vi "Unit Test - copy and Replace State.vi"() -> (3 "Array":T1(array[cluster])=[{"state"="Idle", "error out"={"status"=FALSE, "code"=0, "source"=""}, "Execution:State"=enum."Idle"}, {"state"="CSM Documentation", "error out"={"status"=FALSE, "code"=0, "source"=""}, "Execution:State"=enum."Idle"}, {"state"="VI Reference", "error out"={"status"=FALSE, "code"=0, "source"=""}, "Execution:State"=enum."Idle"}, {"state"="Error Handler", "error out"={"status"=FALSE, "code"=0, "source"=""}, "Execution:State"=enum."Bad"}, {"state"="Critical Error", "error out"={"status"=FALSE, "code"=0, "source"=""}, "Execution:State"=enum."Idle"}, {"state"="Target Timeout Error", "error out"={"status"=FALSE, "code"=0, "source"=""}, "Execution:State"=enum."Idle"}, {"state"="Target Error", "error out"={"status"=FALSE, "code"=0, "source"=""}, "Execution:State"=enum."Idle"}, {"state"="Async Response", "error out"={"status"=FALSE, "code"=0, "source"=""}, "Execution:State"=enum."Idle"}, {"state"="Response", "error out"={"status"=FALSE, "code"=0, "source"=""}, "Execution:State"=enum."Idle"}, {"state"="Async Message Posted", "error out"={"status"=FALSE, "code"=0, "source"=""}, "Execution:State"=enum."Idle"}, {"state"="Initialize Core Data", "error out"={"status"=FALSE, "code"=0, "source"=""}, "Execution:State"=enum."Idle"}, {"state"="Exit", "error out"={"status"=FALSE, "code"=0, "source"=""}, "Execution:State"=enum."Idle"}, {"state"="Data: Initialize", "error out"={"status"=FALSE, "code"=0, "source"=""}, "Execution:State"=enum."Idle"}, {"state"="Data: Update Indicators", "error out"={"status"=FALSE, "code"=0, "source"=""}, "Execution:State"=enum."Idle"}, {"state"="Data: Cleanup", "error out"={"status"=FALSE, "code"=0, "source"=""}, "Execution:State"=enum."Idle"}, {"state"="Macro: Initialize", "error out"={"status"=FALSE, "code"=0, "source"=""}, "Execution:State"=enum."Idle"}, {"state"="Macro: Exit", "error out"={"status"=FALSE, "code"=0, "source"=""}, "Execution:State"=enum."Idle"}, {"state"="API: API1", "error out"={"status"=FALSE, "code"=0, "source"=""}, "Execution:State"=enum."Idle"}, {"state"="API: API2", "error out"={"status"=FALSE, "code"=0, "source"=""}, "Execution:State"=enum."Idle"}, {"state"="Action: action1", "error out"={"status"=FALSE, "code"=0, "source"=""}, "Execution:State"=enum."Idle"}, {"state"="Action: action2", "error out"={"status"=FALSE, "code"=0, "source"=""}, "Execution:State"=enum."Idle"}])   [LabVIEW 2017, in "testcase-csmhelper.lvclass"]
uses:
  testcase-csmhelper.lvclass
  src/user.lib/_NEVSTOP/Communicable State Machine(CSM)/_csmHelper/CSM-Helper.lvclass/CSM-Helper.ctl
  src/user.lib/_NEVSTOP/Communicable State Machine(CSM)/_csmHelper/Properties/Read VI Ref.vi
  src/user.lib/_NEVSTOP/Communicable State Machine(CSM)/_csmHelper/API/Create From VI Reference.vi
  src/user.lib/_NEVSTOP/Communicable State Machine(CSM)/_csmHelper/API/Open Block Diagram.vi
  src/user.lib/_NEVSTOP/Communicable State Machine(CSM)/_csmHelper/Properties/Read User-Defined States.vi
  src/user.lib/_NEVSTOP/Communicable State Machine(CSM)/_csmHelper/API/Start Undo.vi
  src/user.lib/_NEVSTOP/Communicable State Machine(CSM)/_csmHelper/API/Copy State.vi
  src/user.lib/_NEVSTOP/Communicable State Machine(CSM)/_csmHelper/API/Stop Undo.vi
  src/user.lib/_NEVSTOP/Communicable State Machine(CSM)/_csmHelper/API/Undo.vi
  src/user.lib/_NEVSTOP/Communicable State Machine(CSM)/_csmHelper/API/Destroy.vi
  src/user.lib/_NEVSTOP/Communicable State Machine(CSM)/_csmHelper/CSM-Helper.lvclass
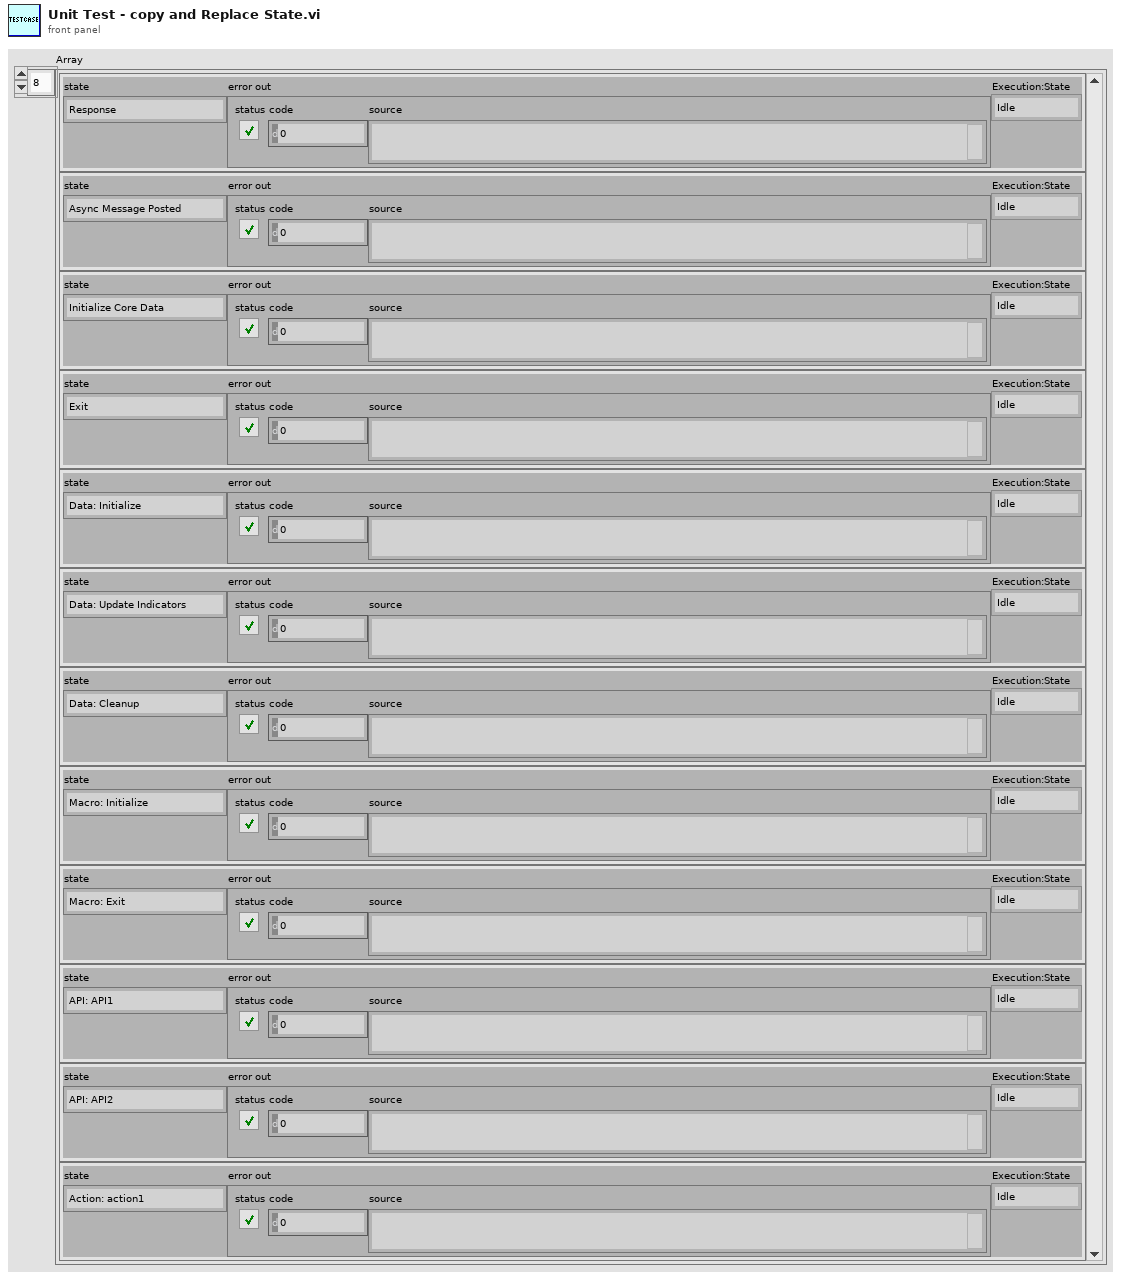
[diagram p1: front panel]
types:
  T1 = cluster{"state":string, "error out":errorcluster, "Execution:State":enum32{"Bad", "Idle", "Run top level", "Running"}}[]
  T2 = enum32{"Bad", "Idle", "Run top level", "Running"}
  T3 = cluster{string, "error out":errorcluster, "Exec.State":enum32{"Bad", "Idle", "Run top level", "Running"}}
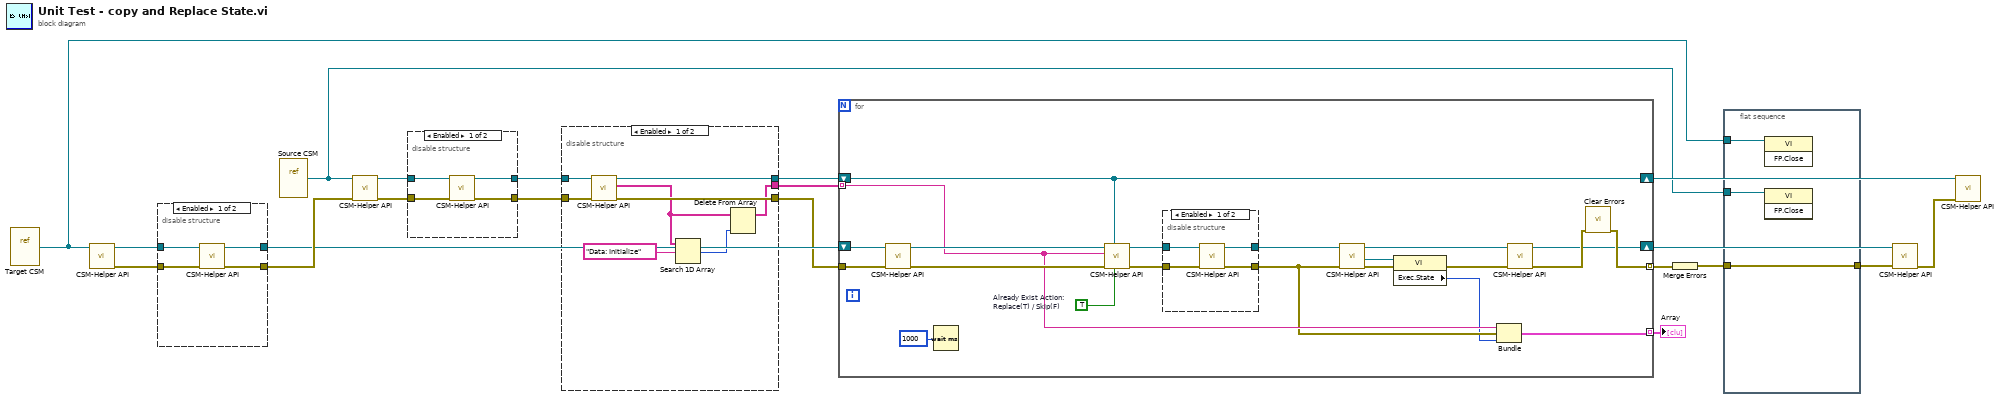
[diagram p0: block diagram]
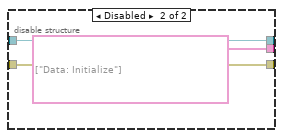
[diagram p2: hidden frame]
diagram:
  n1 = vi-ref "Target CSM.vi"() -> (w2:refnum<vi>)
  n2 = call-poly "CSM-Helper API.vi"("VI"=w2) -> ("error out"=w18:errorcluster, "CSM-Helper.lvclass"=w17:refnum<class "CSM-Helper.lvclass">)  [unwired: 9 in]
  n3 = disable-structure shown="Enabled" {
    disable-tunnel: w18 -> [w24 w26]
    disable-tunnel: w17 -> [w23 w25]
    disable-tunnel: [w22 w26] -> w12
    disable-tunnel: [w21 w25] -> w11
    frame Enabled {
      n4 = call-poly "CSM-Helper API.vi"("error in (no error)"=w24, "CSM-Helper in"=w23) -> ("error out"=w22:errorcluster, "CSM-Helper out"=w21:refnum<class "CSM-Helper.lvclass">)  [unwired: 8 in]
    }
    frame Disabled {
    }
  }
  n5 = vi-ref "Source CSM.vi"() -> (w1:refnum<vi>)
  n6 = call-poly "CSM-Helper API.vi"("error in (no error)"=w12, "VI"=w1) -> ("error out"=w15:errorcluster, "CSM-Helper.lvclass"=w16:refnum<class "CSM-Helper.lvclass">)  [unwired: 8 in]
  n7 = disable-structure shown="Enabled" {
    disable-tunnel: w16 -> [w30 w31]
    disable-tunnel: w15 -> [w29 w32]
    disable-tunnel: [w28 w32] -> w14
    disable-tunnel: [w27 w31] -> w13
    frame Enabled {
      n8 = call-poly "CSM-Helper API.vi"("error in (no error)"=w29, "CSM-Helper in"=w30) -> ("error out"=w28:errorcluster, "CSM-Helper out"=w27:refnum<class "CSM-Helper.lvclass">)  [unwired: 8 in]
    }
    frame Disabled {
    }
  }
  n9 = disable-structure shown="Enabled" {
    disable-tunnel: w14 -> [w40 w42]
    disable-tunnel: w13 -> [w39 w43]
    disable-tunnel: [w38 w42] -> w10
    disable-tunnel: [w37 w43] -> w9
    disable-tunnel: [w34 string[] ["Data: Initialize"] ("Value")] -> w6
    frame Enabled {
      n10 = call-poly "CSM-Helper API.vi"("error in (no error)"=w40, "CSM-Helper in"=w39) -> ("error out"=w38:errorcluster, "Array"=w35:string[], "CSM-Helper out"=w37:refnum<class "CSM-Helper.lvclass">)  [unwired: 7 in]
      n11 = Search 1D Array(1D array=w35, element="Data: Initialize") -> (index of element=w33:i32)  [unwired: 1 in]
      n12 = Delete From Array(array=w35, index=w33) -> (array with subset deleted=w34:string[])  [unwired: 1 in, 1 out]
    }
    frame Disabled {
    }
  }
  n13 = for {
    shift-right: [w52] -> w20
    shift-left: w11 -> [w63]
    shift-right: [w58] -> w7
    shift-left: w9 -> [w58]
    tunnel: w6 -> [w56] mode=indexing
    tunnel: w10 -> [w62]
    tunnel: [w57] -> w19 mode=indexing
    tunnel: [w55] -> w5 mode=indexing
    w44 = TRUE  # Already Exist Action: Replace(T) / Skip(F)
    n14 = call-poly "CSM-Helper API.vi"("error in (no error)"=w62, "CSM-Helper in"=w63) -> ("error out"=w61:errorcluster, "CSM-Helper out"=w60:refnum<class "CSM-Helper.lvclass">)  [unwired: 8 in]
    n15 = Wait (ms)(milliseconds to wait=u32 1000) -> ()  [unwired: 1 out]
    n16 = call-poly "CSM-Helper API.vi"("Already Exist Action:\nReplace(T) / Skip(F)"=w44, "SourceCSM"=w58, "error in (no error)"=w61, "Case"=w56, "CSM-Helper.lvclass"=w60) -> ("error out"=w59:errorcluster, "CSM-Helper out 2"=w64:refnum<class "CSM-Helper.lvclass">)  [unwired: 5 in]
    n17 = disable-structure shown="Enabled" {
      disable-tunnel: [w68 w70] -> w50
      disable-tunnel: w59 -> [w67 w69]
      disable-tunnel: [w66 w69] -> w51
      disable-tunnel: w64 -> [w65 w70]
      frame Enabled {
        n18 = call-poly "CSM-Helper API.vi"("error in (no error)"=w67, "CSM-Helper in"=w65) -> ("error out"=w66:errorcluster, "CSM-Helper out"=w68:refnum<class "CSM-Helper.lvclass">)  [unwired: 8 in]
      }
      frame Disabled {
      }
    }
    n19 = call-poly "CSM-Helper API.vi"("error in (no error)"=w51, "CSM-Helper in"=w50) -> ("error out"=w48:errorcluster, "VI"=w46:refnum<vi>, "CSM-Helper out"=w49:refnum<class "CSM-Helper.lvclass">)  [unwired: 7 in]
    n20 = property class="VI"(reference=w46, error in=w48) -> (error out=w47:errorcluster, "Exec.State"=w45:T2)  [unwired: 1 out]
    n21 = Bundle(w56, "error out"=w51, "Exec.State"=w45) -> (w55:T3)  [unwired: 1 in]
    n22 = call-poly "CSM-Helper API.vi"("error in (no error)"=w47, "CSM-Helper in"=w49) -> ("error out"=w53:errorcluster, "CSM-Helper out"=w52:refnum<class "CSM-Helper.lvclass">)  [unwired: 8 in]
    n23 = call <vilib>:"Clear Errors.vi"("error in (no error)"=w53) -> ("error out"=w57:errorcluster)  [unwired: 5 in, 1 out]
  }
  "Array" <- w5
  n24 = Merge Errors(w19) -> (w4:errorcluster)
  n25 = flat-sequence {
    tunnel: [w73] -> w3
    tunnel: w4 -> [w73]
    tunnel: w1 -> [w72]
    tunnel: w2 -> [w71]
    frame #0 {
      n26 = invoke class="VI" method="FP.Close"(reference=w71) -> ()  [unwired: 2 in, 3 out]
      n27 = invoke class="VI" method="FP.Close"(reference=w72) -> ()  [unwired: 2 in, 3 out]
    }
  }
  n28 = call-poly "CSM-Helper API.vi"("error in (no error)"=w3, "CSM-Helper in"=w20) -> ("error out"=w8:errorcluster)  [unwired: 8 in, 1 out]
  n29 = call-poly "CSM-Helper API.vi"("error in (no error)"=w8, "CSM-Helper in"=w7) -> ()  [unwired: 8 in, 2 out]
